vi "Tenney Adjust Time Interval.vi"(8 "error in (no error)":errorcluster, 10 "Viasala Data Input":T1, 11 "Temperature Limits Input":T2={"Target Temperature Upper limit"=68.0, "Target Temperature Lower limit"=67.0, "Target Humidity Lower limit"=48.5, "Target Humidity Upper limit"=51.5, "Chamber Temperature Upper limit"=68.0, "Chamber Temperature Lower limit"=67.0, "Chamber Humidity Lower limit"=48.5, "Chamber Humidity Upper limit"=51.5, "Chamber Adjustment Increment (F)"=0.1, "Chamber Adjustment Interval (Minutes)"=10.0, "Chamber Adjustment Increment (%)"=0.1, "Chamber Adjustment Interval Fast (Minutes)"=5.0}) -> (0 "error out":errorcluster, 2 "Viasala Data Output":T1, 3 "Temperature Limits Output":T2={"Target Temperature Upper limit"=68.0, "Target Temperature Lower limit"=67.0, "Target Humidity Lower limit"=48.5, "Target Humidity Upper limit"=51.5, "Chamber Temperature Upper limit"=68.0, "Chamber Temperature Lower limit"=67.0, "Chamber Humidity Lower limit"=48.5, "Chamber Humidity Upper limit"=51.5, "Chamber Adjustment Increment (F)"=0.1, "Chamber Adjustment Interval (Minutes)"=10.0, "Chamber Adjustment Increment (%)"=0.1, "Chamber Adjustment Interval Fast (Minutes)"=5.0}, 5 "Increment Selector (0-Normal or 1-Fast)":u8)   [LabVIEW 2023]
uses:
  controls/Tenney Temperature Limits.ctl
  Drivers/Viasala Indigo 520/Type Definitions/Viasala Indigo 520 Data.ctl
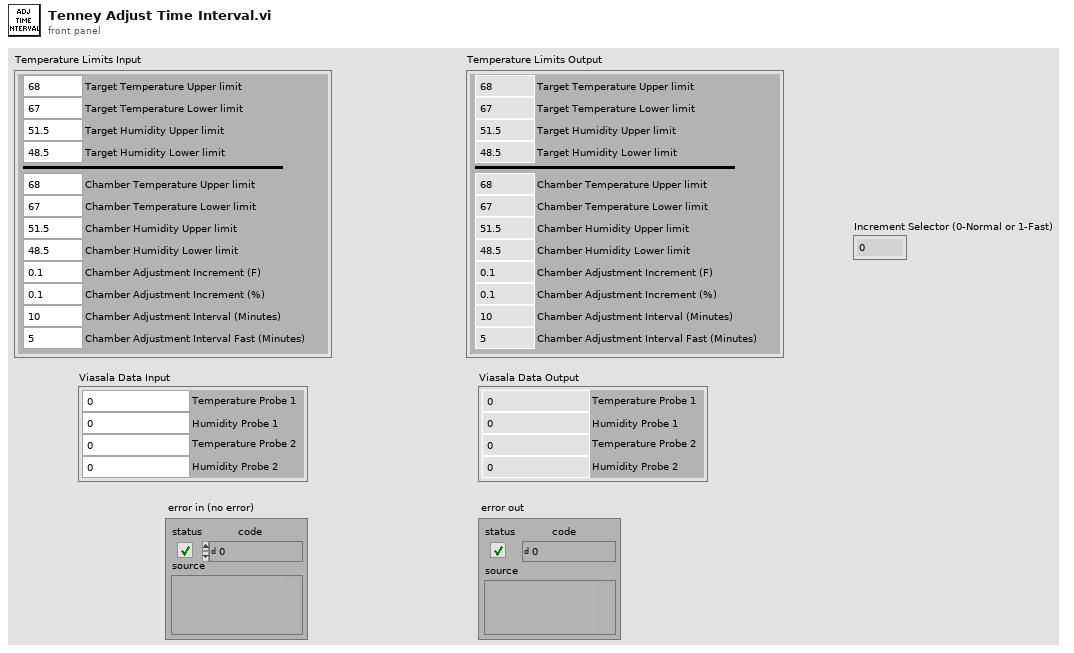
[diagram p1: front panel]
types:
  T1 = typedef "Viasala Indigo 520 Data.ctl" = cluster{"Temperature Probe 1":dbl, "Humidity Probe 1":dbl, "Temperature Probe 2":dbl, "Humidity Probe 2":dbl}
  T2 = typedef "Tenney Temperature Limits.ctl" = cluster{"Target Temperature Upper limit":dbl, "Target Temperature Lower limit":dbl, "Target Humidity Lower limit":dbl, "Target Humidity Upper limit":dbl, "Chamber Temperature Upper limit":dbl, "Chamber Temperature Lower limit":dbl, "Chamber Humidity Lower limit":dbl, "Chamber Humidity Upper limit":dbl, "Chamber Adjustment Increment (F)":dbl, "Chamber Adjustment Interval (Minutes)":dbl, "Chamber Adjustment Increment (%)":dbl, "Chamber Adjustment Interval Fast (Minutes)":dbl}
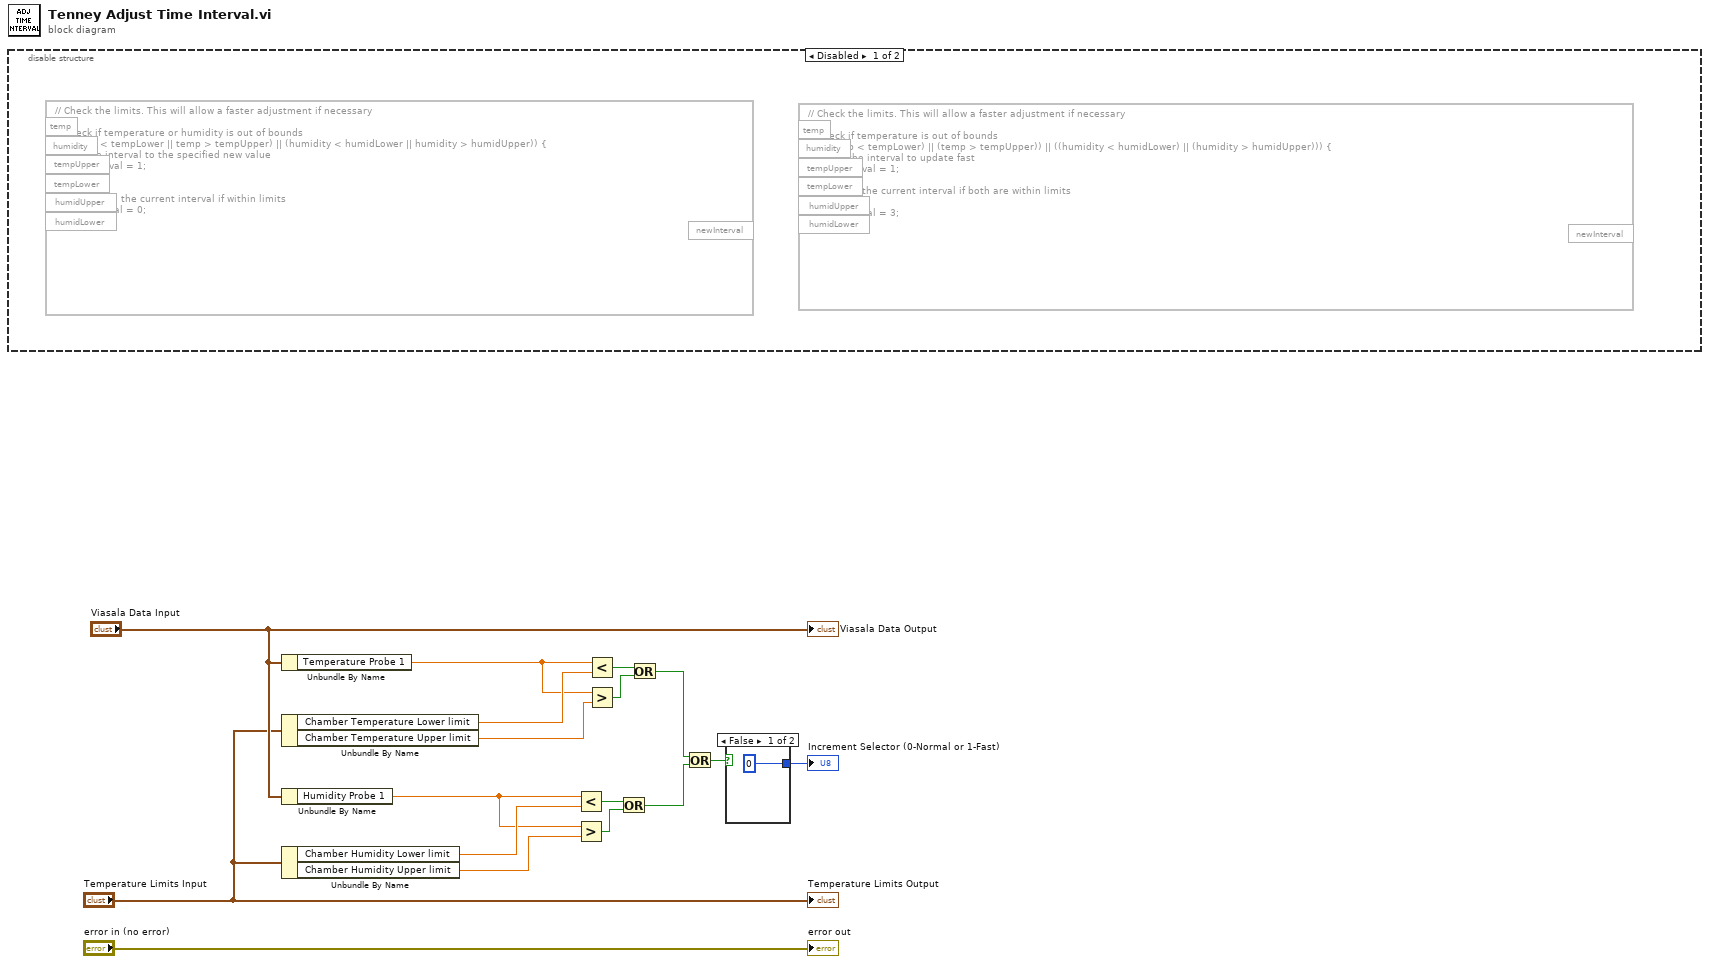
[diagram p0: block diagram]
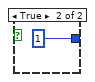
[diagram p2: hidden frame]
diagram:
  n1 = disable-structure shown="Disabled" {
    frame Disabled {
      n2 = formula code="// Check the limits. This will allow a faster adjustment if necessary\n\n// Check if temperature or humidity is out of bounds\nif ((temp < tempLower || temp > tempUpper) || (humidity < humidLower || humidity > humidUpper)) {   \n // Set the interval to the specified new value\n    newInterval = 1;\n} \nelse {\n    // Maintain the current interval if within limits\n    newInterval = 0;\n}"() -> ()  [unwired: 6 in, 1 out]
      n3 = formula code="// Check the limits. This will allow a faster adjustment if necessary\n\n// Check if temperature is out of bounds\nif (((temp < tempLower) || (temp > tempUpper)) || ((humidity < humidLower) || (humidity > humidUpper))) {\n    // Set the interval to update fast\n    newInterval = 1;\n}\n// Maintain the current interval if both are within limits\nelse {\n    newInterval = 3;\n}"() -> ()  [unwired: 6 in, 1 out]
    }
    frame Enabled {
    }
  }
  n4 = Unbundle By Name("Viasala Data Input") -> ("Temperature Probe 1"=w14:dbl)
  n5 = Unbundle By Name("Temperature Limits Input") -> ("Chamber Temperature Lower limit"=w16:dbl, "Chamber Temperature Upper limit"=w13:dbl)
  n6 = Unbundle By Name("Viasala Data Input") -> ("Humidity Probe 1"=w6:dbl)
  n7 = Unbundle By Name("Temperature Limits Input") -> ("Chamber Humidity Lower limit"=w7:dbl, "Chamber Humidity Upper limit"=w5:dbl)
  n8 = Less?(x=w6, y=w7) -> (x < y?=w8:bool)
  n9 = Greater?(x=w6, y=w5) -> (0:w9:bool)
  n10 = Less?(x=w14, y=w16) -> (x < y?=w15:bool)
  n11 = Greater?(x=w14, y=w13) -> (0:w12:bool)
  n12 = Or(x=w8, y=w9) -> (x .or. y?=w3:bool)
  n13 = Or(x=w15, y=w12) -> (x .or. y?=w4:bool)
  n14 = Or(x=w4, y=w3) -> (x .or. y?=w2:bool)
  n15 = case shown="False" w2 {
    tunnel: [u8 0 ("Increment Selector (0-Normal or 1-Fast)") u8 1 ("Increment Selector (0-Normal or 1-Fast)")] -> w1
    frame False {
    }
    frame True {
    }
  }
  "Increment Selector (0-Normal or 1-Fast)" <- w1
  "error out" <- "error in (no error)"
  "Viasala Data Output" <- "Viasala Data Input"
  "Temperature Limits Output" <- "Temperature Limits Input"
